vi "Configure Marker Frequency.vi"(8 "error in (no error)":errorcluster, 9 "Marker Number (1)":u32=1 min=1, 10 "Marker Frequency [Hz]":dbl, 11 "SA-ESA in":refnum<class "SA-ESA.lvclass">) -> (0 "error out":errorcluster, 3 "SA-ESA out":refnum<class "SA-ESA.lvclass">)   [LabVIEW 2020, in "SA-ESA.lvclass"]
uses:
  SA-ESA.lvclass
  C:/Sandbox/Git_Sandbox/WiSpry Test Framework source code (LV20)/WiSpry Test Framework/Instruments/Instrument.lvclass
  Instrument.lvclass/Instrument.ctl
  Instrument.lvclass
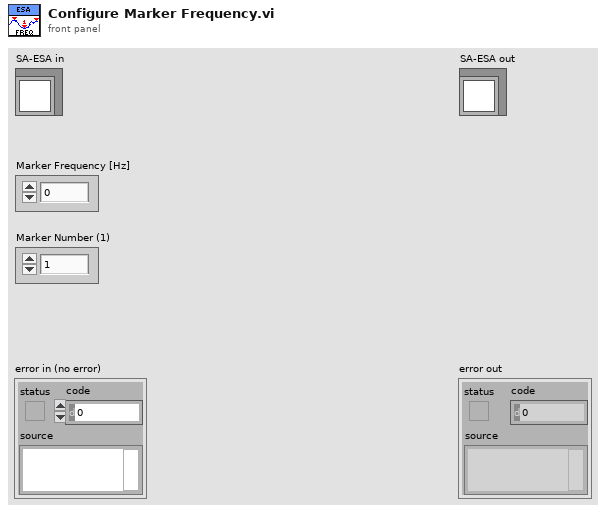
[diagram p1: front panel]
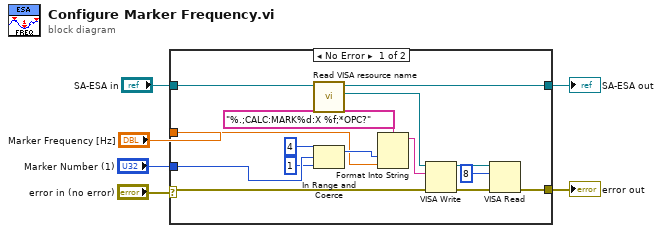
[diagram p0: block diagram]
diagram:
  n1 = case shown="No Error" "error in (no error)" {
    selector: "error in (no error)" -> [w12 w22]
    tunnel: "SA-ESA in" -> [w21 w23]
    tunnel: "Marker Number (1)" -> [w20 _]
    tunnel: "Marker Frequency [Hz]" -> [w16 _]
    tunnel: [w8 w23] -> w2
    tunnel: [w7 w22] -> w1
    frame No Error {
      n2 = call "Read VISA resource name.vi"("Instrument in"=w21) -> ("VISA resource name"=w14:refnum<visa-resource-name>, "Instrument out"=w8:refnum<class "SA-ESA.lvclass">)  [unwired: 9 in]
      n3 = In Range and Coerce(upper limit=u32 4, x=w20, lower limit=u32 1) -> (coerced(x)=w17:u32)  [unwired: 1 out]
      n4 = Format Into String(format string="%.;CALC:MARK%d:X %f;*OPC?", w17, w16) -> (resulting string=w13:string)  [unwired: 2 in, 1 out]
      n5 = VISA Write(VISA resource name=w14, write buffer=w13, error in (no error)=w12) -> (VISA resource name out=w11:refnum<visa-resource-name>, error out=w10:errorcluster)  [unwired: 1 out]
      n6 = VISA Read(VISA resource name=w11, byte count=u32 8, error in (no error)=w10) -> (error out=w7:errorcluster)  [unwired: 3 out]
    }
    frame Error {
    }
  }
  "error out" <- w1
  "SA-ESA out" <- w2
